vi "Waveform.vi"() -> ()   [LabVIEW 2023]
panel:
  in  "Connect":bool
  in  "CLOSE":bool
  in  "WRITE":bool
  in  "Command IN":string
  in  "VISA Refnum in":refnum<visa-resource-name>
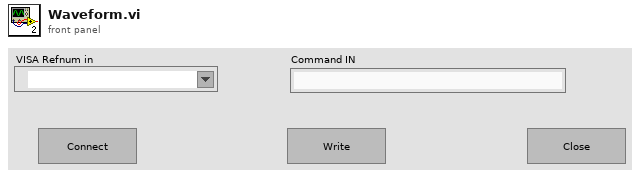
[diagram p1: front panel]
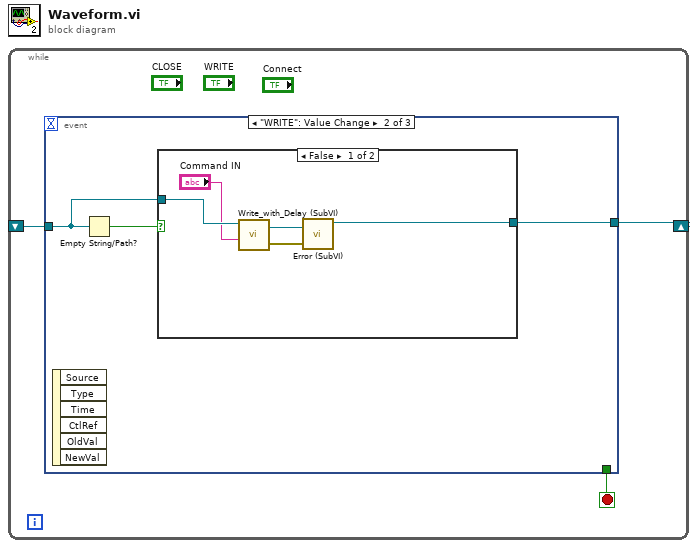
[diagram p0: block diagram]
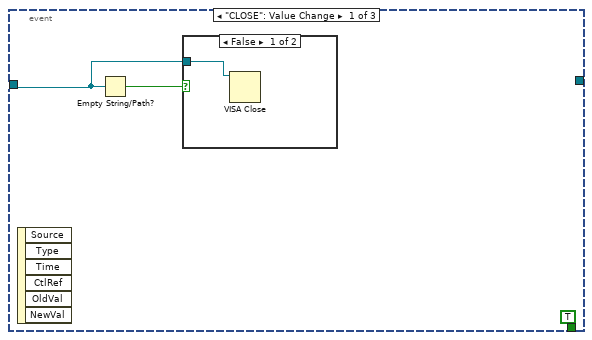
[diagram p2: hidden frame]
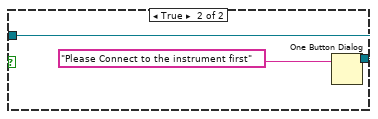
[diagram p4: hidden frame]
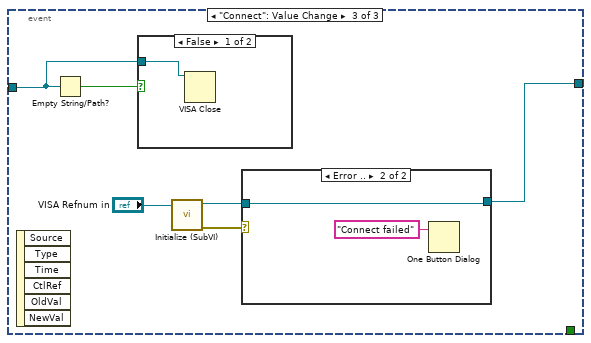
[diagram p5: hidden frame]
diagram:
  n1 = while {
    shift-right: [w1] -> _
    shift-left: _ -> [w2]
    stop <- w3 stop-if-true
    n2 = event shown="[1] \"WRITE\": Value Change" {
      selector: _ -> [_ _ _]
      dyn-events: _ -> [_ _ _]
      timeout: _ -> [_ _ _]
      tunnel: [TRUE _ _] -> w3
      tunnel: w2 -> [w4 w9 w22]
      tunnel: [_ w8 w21] -> w1
      event "CLOSE": Value Change {
        n3 = event-data() -> ()  [unwired: 1 in, 6 out]
        n4 = Empty String/Path?(string/path=w4) -> (empty?=w5:bool)
        n5 = case shown="False" w5 {
          tunnel: w4 -> [w7 _]
          frame False {
            n6 = VISA Close(VISA resource name=w7) -> ()  [unwired: 1 in, 1 out]
          }
          frame True {
          }
        }
      }
      event "WRITE": Value Change {
        n7 = event-data() -> ()  [unwired: 1 in, 6 out]
        n8 = Empty String/Path?(string/path=w9) -> (empty?=w10:bool)
        n9 = case shown="False" w10 {
          tunnel: w9 -> [w15 w16]
          tunnel: [w11 w16] -> w8
          frame False {
            n10 = call "Write_with_Delay (SubVI).vi"("Command"="Command IN", "VISA Refnum in"=w15) -> ("error out"=w12:errorcluster, "VISA Refnum out"=w13:refnum<visa-resource-name>)  [unwired: 2 in]
            n11 = call "Error (SubVI).vi"("error in (no error)"=w12, "VISA Refnum in"=w13) -> ("VISA Refnum out"=w11:refnum<visa-resource-name>)  [unwired: 6 in, 3 out]
          }
          frame True {
            n12 = One Button Dialog(message="Please Connect to the instrument first") -> ()  [unwired: 1 in, 1 out]
          }
        }
      }
      event "Connect": Value Change {
        n13 = event-data() -> ()  [unwired: 1 in, 6 out]
        n14 = Empty String/Path?(string/path=w22) -> (empty?=w23:bool)
        n15 = case shown="False" w23 {
          tunnel: w22 -> [w27 _]
          frame False {
            n16 = VISA Close(VISA resource name=w27) -> ()  [unwired: 1 in, 1 out]
          }
          frame True {
          }
        }
        n17 = call "Initialize (SubVI).vi"("VISA Refnum in"="VISA Refnum in") -> ("error out"=w18:errorcluster, "VISA Refnum out"=w19:refnum<visa-resource-name>)  [unwired: 9 in]
        n18 = case shown="Error .." w18 {
          tunnel: w19 -> [w24 w25]
          tunnel: [w24 w25] -> w21
          frame No Error {
          }
          frame Error {
            n19 = One Button Dialog(message="Connect failed") -> ()  [unwired: 1 in, 1 out]
          }
        }
      }
    }
  }
